vi "Untitled 1-save me.vi"() -> ()   [LabVIEW 2011]
uses:
  <vilib>/DAQmx/read.llb/DAQmx Read (Analog Wfm 1Chan NSamp).vi
  <vilib>/DAQmx/create/channels.llb/DAQmx Create Channel (AI-Current-Basic).vi
  <vilib>/DAQmx/configure/timing.llb/DAQmx Timing (Sample Clock).vi
  <vilib>/DAQmx/miscellaneous.llb/DAQmx Fill In Error Info.vi
  <vilib>/Analysis/NI_AALBase.lvlib
panel:
  in  "ECOLAB Button":bool=TRUE
  out "Max Value":dbl
  out "Maximum":string
  out "Block Count":i32
  in  "Tab Control":enum32{"DISPLAY", "CONFIG", "CALIBRATE"}(tab)
  in  "Intervals":i32=10
  in  "Rate (Inches / Second)":dbl
  out "XY Graph":cluster{dbl[], "Initialize Value":dbl[]}(graph)
  out "Histogram Graph":T1(graph)
  out "Save Error":errorcluster
  out "Distance Between Measurements (Inches)":dbl
  out "dt":dbl
  out "Main Error":errorcluster
  out "DAQ Error":errorcluster
  in  "DAQ Selection":tag
  in  "File Path Input":path
  in  "Samples/Channel":i32=5
  in  "Sample Rate (Hz)":dbl=500.0
  in  "Comments (Saves to Data File)":string
  in  "Scale Template":T2={"Channel Select"=0, "Clear/Reset Scales"=FALSE, "Channel #"=["0", "1", "2"], "Scale Names"=["a", "b", "c"], "Set?"=[FALSE, FALSE, FALSE, FALSE, FALSE, FALSE], "HI/LO Setpoints"=[1.0, 0.0, 1.0, 0.0, 1.0, 0.0], "Units"=["vdc", "vdc", "vdc"], "HI/LO Signals"=[1.0, 0.0, 1.0, 0.0, 1.0, 0.0], "Slope/Intercept"=[1.0, 0.0, 1.0, 0.0, 1.0, 0.0], "IN/OUT Values"=[1.0, 1.0, 2.0, 2.0, 3.0, 3.0]} {"Channel Select" min=0 step=1; "Slope/Intercept" format="%#.3p"; "HI/LO Setpoints" format="%#.3p"; "IN/OUT Values" format="%#.3p"; "HI/LO Signals" format="%#.3p"}
  in  "Simulate Signal?":bool
  in  "Simulated Signal":dbl
  in  "Stop Program":bool
  out "Measurements 2":string[](array[string])
  in  "Analyze Data?":bool
  in  "Reset Block Count?":bool
  in  "Update Rate [ms] 2":u32
  out "DAQ Loop":i32
  in  "Distance Threshold (> = Measure)":dbl
  in  "Save Data Signal":bool
  in  "Update Rate [ms]":u32
  in  "Input Signal":dbl
  in  "Flow Volume":dbl
  in  "Reset Spray Count":bool
  out "Spray Count":i32
  out "Temperature OUT":cluster{"Mean":dbl, "Stdev":dbl, "Max":dbl}
  out "output array":dbl[](array[numeric])
  out "Flow Delta":dbl
  out "loop":i32
  in  "stop":bool
  in  "Spray Signal":bool=TRUE
  # "Threshold (inches)"
  # "Block Count"
  # "Maximum (inches)"
  # "Block Profile Measurement Program"
  # "Blake Otting - 2011"
  # "Histogram of Maximum Value Measurements"
  # "Measurement Profile of Last Block"
  # "Track Rate"
  # "Inches / Second"
  # "Ch.\n#"
  # "Scale\nName"
  # "Set\nValues?"
  # "Scaled"
  # "Pre-Scaled"
  # "Scaling Result"
  # "Values"
  # "Units"
  # "Values"
  # "Channel\nSelect"
  # "HI"
  # "Slope"
  # "IN"
  # "LO"
  # "Intercept"
  # "OUT"
  # "HI"
  # "Slope"
  # "IN"
  # "LO"
  # "Intercept"
  # "OUT"
  # "HI"
  # "Slope"
  # "IN"
  # "LO"
  # "Intercept"
  # "OUT"
  # "HI"
  # "Slope"
  # "IN"
  # "LO"
  # "Intercept"
  # "OUT"
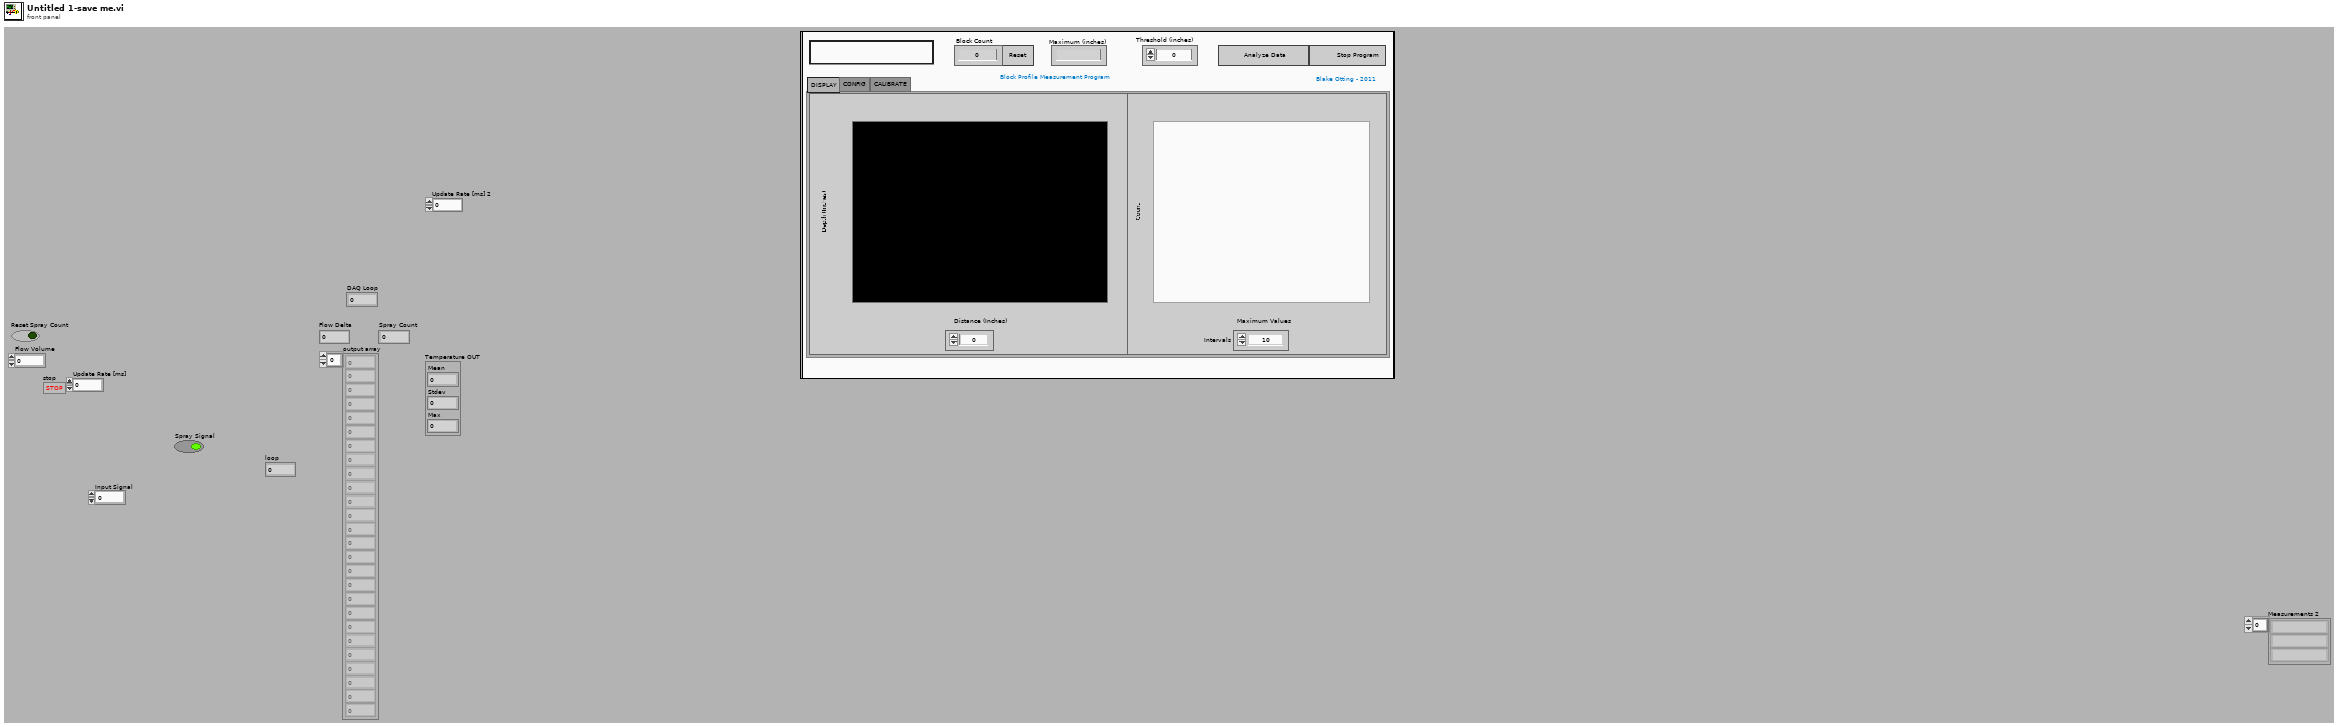
[diagram p1: front panel]
types:
  T1 = cluster{"X Values":dbl[], "Histogram: h(x)":i32[]}
  T2 = cluster{"Channel Select":i32, "Clear/Reset Scales":bool, "Channel #":string[], "Scale Names":string[], "Set?":bool[], "HI/LO Setpoints":dbl[], "Units":string[], "HI/LO Signals":dbl[], "Slope/Intercept":dbl[], "IN/OUT Values":dbl[]}
  T3 = cluster{"Delta":dbl, "Mean":dbl, "Stdev":dbl, "Max":dbl}
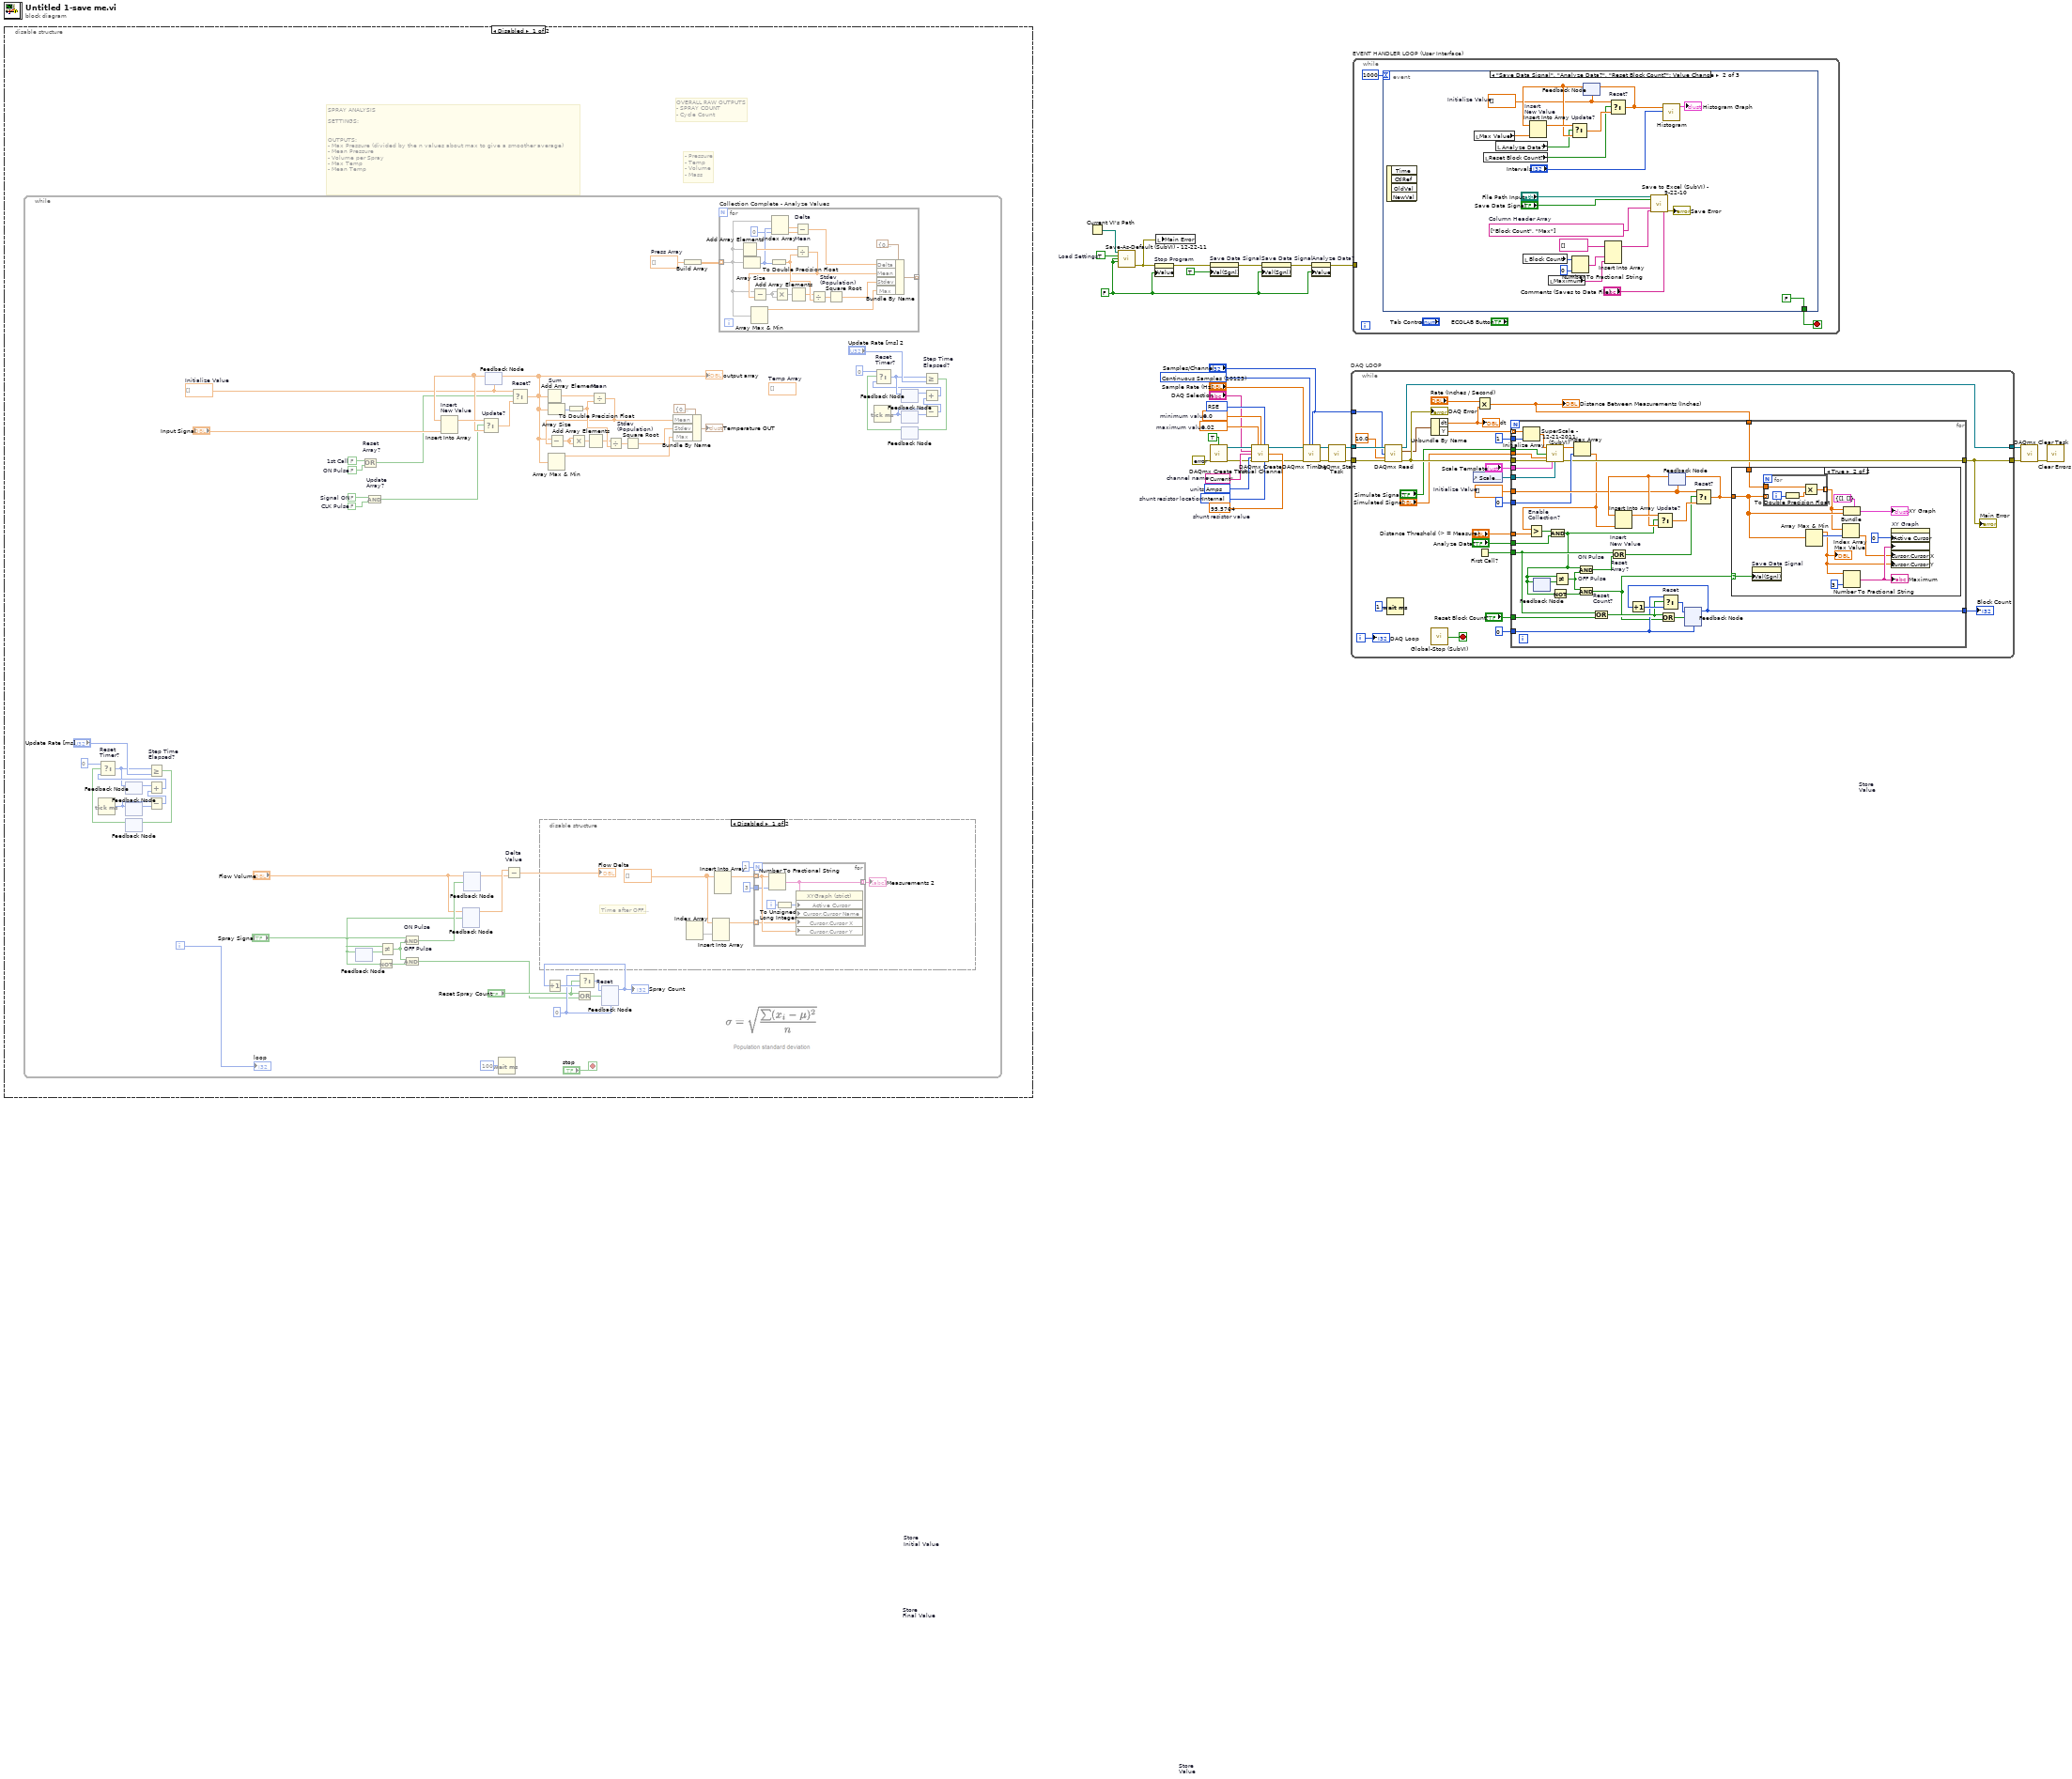
[diagram p0: block diagram]
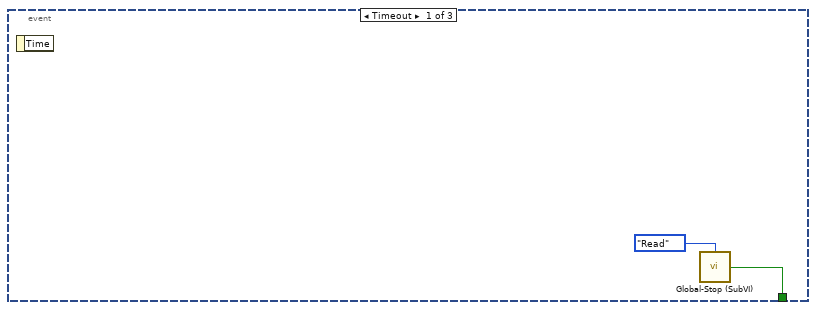
[diagram p2: hidden frame]
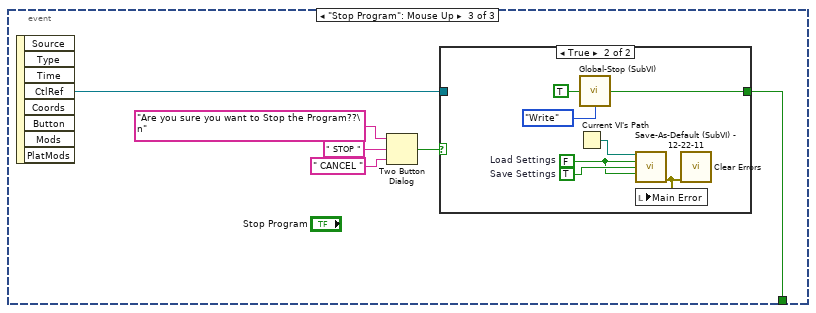
[diagram p3: hidden frame]
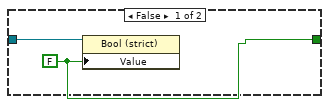
[diagram p4: hidden frame]
diagram:
  w5 = TRUE  # Load Settings
  w3 = FALSE
  w17 = 10123 items=["Finite Samples"=10178, "Continuous Samples"=10123, "Hardware Timed Single Point"=12522] ("Sample Mode")
  w25 = 10083 items=["default"=-1, "RSE"=10083, "NRSE"=10078, "Differential"=10106, "Pseudodifferential"=12529]
  w26 = 10342 items=["Amps"=10342, "From Custom Scale"=10065]  # units
  w27 = 95.5764  # shunt resistor value
  w28 = 10200 items=["Internal"=10200, "External"=10167]  # shunt resistor location
  w29 = "Current"  # channel name
  w30 = 0.0  # minimum value
  w31 = 0.02  # maximum value
  n1 = disable-structure shown="Disabled" {
    frame Disabled {
      # "- Pressure\n- Temp\n- Volume\n- Mass"
      # "OVERALL RAW OUTPUTS\n- SPRAY COUNT\n- Cycle Count"
      # "SPRAY ANALYSIS\n\nSETTINGS:\n\n\nOUTPUTS:\n- Max Pressure (divided by the n values about max to give a smoother average)\n- Mean Pressure\n- Volume per Spray \n- Max Temp\n- Mean Temp"
      n2 = while {
        i -> [w90]
        stop <- "stop" stop-if-true
        w46 = FALSE  # CLK Pulse
        w47 = FALSE  # Signal ON
        w49 = FALSE  # ON Pulse
        w50 = FALSE  # 1st Call
        w62 = dbl[] []  # Initialize Value
        w71 = 0 ("index")
        w75 = dbl[] []  # Press Array
        (unwired) dbl[] []  # Temp Array
        # "Time after OFF..."
        n3 = Tick Count (ms)() -> (millisecond timer value=w58:u32)
        n4 = feedback #1() -> (w59:u32)  [unwired: 1 in]
        n5 = feedback #2() -> (w57:u32)  [unwired: 1 in]
        n6 = feedback-in #2(w58) -> ()
        n7 = feedback #3() -> (w52:bool)  [unwired: 1 in]
        n8 = Subtract(x=w58, y=w57) -> (x-y=w55:u32)
        n9 = Add(x=w59, y=w55) -> (x+y=w60:u32)
        n10 = Select "Reset\nTimer?"(t=u32 0 ("x+y"), s=w52, f=w60) -> (s? t:f=w51:u32)
        n11 = feedback-in #1(w51) -> ()
        n12 = Greater Or Equal? "Step Time\nElapsed?"(x=w51, y="Update Rate [ms]") -> (x >= y?=w53:bool)
        n13 = feedback-in #3(w53) -> ()
        n14 = feedback #4() -> (w98:bool)  [unwired: 1 in]
        n15 = feedback-in #4("Spray Signal") -> ()
        n16 = Or "Reset\nArray?"(x=w50, y=w49) -> (x .or. y?=w48:bool)
        n17 = And "Update\nArray?"(x=w47, y=w46) -> (x .and. y?=w45:bool)
        n18 = Not(x="Spray Signal") -> (.not. x?=w94:bool)
        n19 = Not Equal?(x="Spray Signal", y=w98) -> (x != y?=w95:bool)
        n20 = And "ON Pulse"(x="Spray Signal", y=w95) -> (x .and. y?=w89:bool)
        n21 = And "OFF Pulse"(x=w95, y=w94) -> (x .and. y?=w67:bool)
        n22 = feedback #5 "Store \nFinal Value"() -> (w93:dbl)  [unwired: 1 in]
        n23 = feedback-in #5("Flow Volume", "Spray Signal") -> ()
        n24 = feedback #6 "Store \nInitial Value"() -> (w92:dbl)  [unwired: 1 in]
        n25 = feedback-in #6("Flow Volume", w89) -> ()
        n26 = feedback #7(w62) -> (w64:dbl[])
        n27 = Insert Into Array "Insert \nNew Value"(array=w64, new element="Input Signal") -> (w65:dbl[])  [unwired: 1 in]
        n28 = Select "Update?"(t=w65, s=w45, f=w64) -> (s? t:f=w63:dbl[])
        n29 = Wait (ms)(milliseconds to wait=u32 100) -> ()  [unwired: 1 out]
        n30 = Subtract "Delta\nValue"(x=w93, y=w92) -> (x-y=→"Flow Delta":dbl)
        n31 = Select "Reset?"(t=w62, s=w48, f=w63) -> (s? t:f=w44:dbl[])
        "output array" <- w44
        n32 = feedback-in #7(w44) -> ()
        n33 = disable-structure shown="Disabled" {
          frame Disabled {
            w104 = dbl[] [] ("appended array")
            n34 = Index Array() -> (element #1=w105, index #1=w110:i32, element #2=w103, index #2=w109:i32)  [unwired: 1 in]
            n35 = Insert Into Array(array=w104, new element #1=w105, new element #2=w103) -> (w102:dbl[])  [unwired: 1 in]
            n36 = Insert Into Array(array=w104) -> (w107:dbl[], new element #1=w108:dbl, new element #2=w106:dbl)  [unwired: 1 in]
            n37 = for {
              N: 1 -> [_]
              tunnel: [w114] -> w99 mode=indexing
              tunnel: w107 -> [w113] mode=indexing
              tunnel: w102 -> [w112] mode=indexing
              tunnel: i16 3 ("precision (6)") -> [w111]
              i -> [w115]
              n38 = Number To Fractional String(number=w113, precision (6)=w111) -> (F-format string=w114:string)  [unwired: 2 in]
              n39 = To Unsigned Long Integer(number=w115) -> (unsigned 32bit integer=w116:u32)
              n40 = property on="Property Node" class="XYGraph (strict)"("Active Cursor"=w116, "Cursor.Cursor Name"=w114, "Cursor.Cursor X"=w112, "Cursor.Cursor Y"=w113) -> ()  [unwired: 2 in, 2 out]
            }
            "Measurements 2" <- w99
          }
          frame Enabled {
          }
        }
        n41 = Add Array Elements "Sum"(numeric array=w44) -> (sum=w87:dbl)
        n42 = Array Size(array=w44) -> (size(s)=w86:i32)
        n43 = Array Max & Min(array=w44) -> (max value=w78:dbl)  [unwired: 3 out]
        n44 = To Double Precision Float(number=w86) -> (double precision float=w83:dbl)
        n45 = Or(x="Reset Spray Count", y=w67) -> (x .or. y?=w68:bool)
        n46 = Divide "Mean"(x=w87, y=w83) -> (x/y=w77:dbl)
        n47 = Subtract(x=w44, y=w77) -> (x-y=w85:dbl[])
        n48 = Multiply(x=w85, y=w85) -> (x*y=w84:dbl[])
        n49 = Add Array Elements(numeric array=w84) -> (sum=w82:dbl)
        n50 = feedback #8 "Store\nValue"(w71) -> (w73:i32)
        "Spray Count" <- w73
        n51 = Increment(x=w73) -> (x+1=w72:i32)
        n52 = Select "Reset"(t=w71, s="Reset Spray Count", f=w72) -> (s? t:f=w70:i32)
        n53 = feedback-in #8(w70, w68) -> ()
        n54 = Divide(x=w82, y=w83) -> (x/y=w81:dbl)
        n55 = Square Root "Stdev\n(Population)"(x=w81) -> (sqrt(x)=w79:dbl)
        n56 = Bundle By Name(cluster=cluster{"Mean":dbl, "Stdev":dbl, "Max":dbl} {"Mean"=0.0, "Stdev"=0.0, "Max"=0.0}, "Mean"=w77, "Stdev"=w79, "Max"=w78) -> (→"Temperature OUT":cluster{"Mean":dbl, "Stdev":dbl, "Max":dbl})
        n57 = Build Array(w75) -> (w74:dbl[][])
        n58 = for "Collection Complete - Analyze Values" {
          tunnel: w74 -> [w118] mode=indexing
          tunnel: [w117] -> _ mode=indexing
          n59 = Add Array Elements(numeric array=w118) -> (sum=w133:dbl)
          n60 = Array Size(array=w118) -> (size(s)=w123:i32)
          n61 = Array Max & Min(array=w118) -> (max value=w125:dbl)  [unwired: 3 out]
          n62 = To Double Precision Float(number=w123) -> (double precision float=w130:dbl)
          n63 = Index Array(array=w118, index #1=w123, index #2=0 ("index")) -> (element #1=w120:dbl, element #2=w121:dbl)
          n64 = Subtract "Delta"(x=w120, y=w121) -> (x-y=w119:dbl)
          n65 = Divide "Mean"(x=w133, y=w130) -> (x/y=w124:dbl)
          n66 = Subtract(x=w118, y=w124) -> (x-y=w132:dbl[])
          n67 = Multiply(x=w132, y=w132) -> (x*y=w131:dbl[])
          n68 = Add Array Elements(numeric array=w131) -> (sum=w129:dbl)
          n69 = Divide(x=w129, y=w130) -> (x/y=w128:dbl)
          n70 = Square Root "Stdev\n(Population)"(x=w128) -> (sqrt(x)=w126:dbl)
          n71 = Bundle By Name(cluster=T3 {"Delta"=0.0, "Mean"=0.0, "Stdev"=0.0, "Max"=0.0}, "Delta"=w119, "Mean"=w124, "Stdev"=w126, "Max"=w125) -> (w117:T3)
        }
        n72 = Tick Count (ms)() -> (millisecond timer value=w42:u32)
        n73 = feedback #9() -> (w43:u32)  [unwired: 1 in]
        n74 = feedback #10() -> (w41:u32)  [unwired: 1 in]
        n75 = feedback-in #10(w42) -> ()
        n76 = feedback #11() -> (w36:bool)  [unwired: 1 in]
        n77 = Subtract(x=w42, y=w41) -> (x-y=w39:u32)
        n78 = Add(x=w43, y=w39) -> (x+y=w34:u32)
        n79 = Select "Reset\nTimer?"(t=u32 0 ("x+y"), s=w36, f=w34) -> (s? t:f=w35:u32)
        n80 = feedback-in #9(w35) -> ()
        n81 = Greater Or Equal? "Step Time\nElapsed?"(x=w35, y="Update Rate [ms] 2") -> (x >= y?=w37:bool)
        n82 = feedback-in #11(w37) -> ()
        "loop" <- w90
      }
    }
    frame Enabled {
    }
  }
  n83 = Current VI's Path() -> (path=w6:path)
  n84 = call "Save-As-Default (SubVI) - 12-22-11.vi"("Current VI's Path"=w6, "Load Settings"=w5, "Save Settings"=w3, "Save and Exit"=w3) -> ("Error Output"=w4:errorcluster)  [unwired: 11 in]
  n85 = property on="Stop Program" class="Bool (strict)"(error in=w4, "Value"=w3) -> (error out=w7:errorcluster)  [unwired: 1 in, 1 out]
  n86 = local write "Main Error"(w4) -> ()
  n87 = property on="Save Data Signal" class="Bool (strict)"(error in=w7, "Val(Sgnl)"=TRUE) -> (error out=w8:errorcluster)  [unwired: 1 in, 1 out]
  n88 = call <vilib>:"DAQmx Create Task.vi"("auto cleanup"=TRUE, "error in"=errorcluster {"status"=FALSE, "code"=0, "source"=""}) -> ("task out"=w24:refnum<k21>, "error out"=w23:errorcluster)  [unwired: 12 in]
  n89 = call-poly <vilib>:"DAQmx Create Virtual Channel.vi"("task in"=w24, "maximum value"=w31, "minimum value"=w30, "input terminal configuration"=w25, "physical channels"="DAQ Selection", "name to assign"=w29, "external shunt resistor value"=w27, "units"=w26, "error in"=w23, "shunt resistor location"=w28) -> ("task out"=w16:refnum<k21>, "error out"=w15:errorcluster)  [unwired: 1 in, 3 out]
  n90 = property on="Save Data Signal" class="Bool (strict)"(error in=w8, "Val(Sgnl)"=w3) -> (error out=w2:errorcluster)  [unwired: 1 in, 1 out]
  n91 = call-poly <vilib>:"DAQmx Timing.vi"("task/channels in"=w16, "sample mode"=w17, "samples per channel"="Samples/Channel", "rate"="Sample Rate (Hz)", "error in"=w15) -> ("task out"=w13:refnum<k21>, "error out"=w14:errorcluster)  [unwired: 2 in, 7 out]
  n92 = property on="Analyze Data?" class="Bool (strict)"(error in=w2, "Value"=w3) -> (error out=w1:errorcluster)  [unwired: 1 in, 1 out]
  n93 = call <vilib>:"DAQmx Start Task.vi"("task/channels in"=w13, "error in"=w14) -> ("task out"=w12:refnum<k21>, "error out"=w11:errorcluster)  [unwired: 12 in]
  n94 = while "DAQ LOOP" {
    tunnel: [w134] -> w32
    tunnel: w11 -> [w147]
    tunnel: w12 -> [w148]
    tunnel: [w138] -> w19
    tunnel: "Samples/Channel" -> [w146]
    i -> [w161]
    stop <- w139 stop-if-true
    w149 = dbl[] []  # Initialize Value
    n95 = call-poly <vilib>:"DAQmx Read.vi"("task/channels in"=w148, "number of samples per channel"=w146, "timeout"=10.0, "error in"=w147) -> ("task out"=w134:refnum<k21>, "data"=w143:waveform(dbl), "error out"=w144:errorcluster)  [unwired: 9 in]
    "DAQ Error" <- w144
    n96 = Wait (ms)(milliseconds to wait=u32 1) -> ()  [unwired: 1 out]
    n97 = Unbundle By Name(w143) -> ("dt"=w141:dbl, "Y"=w142:dbl[])
    "dt" <- w141
    n98 = call "Global-Stop (SubVI).vi"() -> ("OUT"=w139:bool)  [unwired: 4 in]
    n99 = control-ref of="Scale Template"() -> (w155:refnum<vi>)
    n100 = Multiply(x="Rate (Inches / Second)", y=w141) -> (x*y=w135:dbl)
    "Distance Between Measurements (Inches)" <- w135
    n101 = First Call?() -> (First Call?: T/F=w153:bool)
    n102 = for {
      tunnel: w142 -> [w197] mode=indexing
      tunnel: "Distance Threshold (> = Measure)" -> [w165]
      tunnel: "Analyze Data?" -> [w181]
      tunnel: w149 -> [w180]
      tunnel: 1 ("dimension size") -> [w178]
      tunnel: 0 ("index") -> [w177]
      tunnel: 0 ("index") -> [w176]
      tunnel: w153 -> [w175]
      tunnel: "Reset Block Count?" -> [w174]
      tunnel: [w173] -> w138
      tunnel: w144 -> [w172]
      tunnel: "Scale Template" -> [w171]
      tunnel: w155 -> [w170]
      tunnel: [w167] -> w156
      tunnel: w135 -> [w168]
      tunnel: "Simulate Signal?" -> [w164]
      tunnel: "Simulated Signal" -> [w163]
      n103 = Initialize Array(w197, w178) -> (w196:dbl[])
      n104 = feedback #12() -> (w189:bool)  [unwired: 1 in]
      n105 = call "SuperScale - 12-21-2011 (SubVI).vi"("Measured Signals"=w196, "Simulate Signal?"=w164, "Simulated Signal"=w163, "Error Input"=w172, "Scale Template"=w171, "Scale Ref"=w170) -> ("Scaled Values"=w195:dbl[], "Scale Error"=w173:errorcluster)  [unwired: 8 in]
      n106 = Index Array(array=w195, index=w177) -> (element=w169:dbl)
      n107 = Greater? "Enable\nCollection?"(x=w169, y=w165) -> (0:w194:bool)
      n108 = And(x=w194, y=w181) -> (x .and. y?=w162:bool)
      n109 = feedback-in #12(w162) -> ()
      n110 = Not(x=w162) -> (.not. x?=w187:bool)
      n111 = Not Equal?(x=w162, y=w189) -> (x != y?=w188:bool)
      n112 = And "ON Pulse"(x=w162, y=w188) -> (x .and. y?=w183:bool)
      n113 = And "OFF Pulse"(x=w188, y=w187) -> (x .and. y?=w166:bool)
      n114 = Or "Reset\nCount?"(x=w175, y=w174) -> (x .or. y?=w182:bool)
      n115 = Or "Reset\nArray?"(x=w175, y=w183) -> (x .or. y?=w190:bool)
      n116 = Or(x=w182, y=w166) -> (x .or. y?=w184:bool)
      n117 = feedback #13(w180) -> (w192:dbl[])
      n118 = Insert Into Array "Insert \nNew Value"(array=w192, new element=w169) -> (w193:dbl[])  [unwired: 1 in]
      n119 = Select "Update?"(t=w193, s=w162, f=w192) -> (s? t:f=w191:dbl[])
      n120 = feedback #14 "Store\nValue"(w176) -> (w167:i32)
      n121 = Increment(x=w167) -> (x+1=w186:i32)
      n122 = Select "Reset"(t=w176, s=w182, f=w186) -> (s? t:f=w185:i32)
      n123 = feedback-in #14(w185, w184) -> ()
      n124 = Select "Reset?"(t=w180, s=w190, f=w191) -> (s? t:f=w179:dbl[])
      n125 = feedback-in #13(w179) -> ()
      n126 = case shown="True" w166 {
        selector: w166 -> [_ w198]
        tunnel: w179 -> [_ w208]
        tunnel: w168 -> [_ w209]
        frame False {
        }
        frame True {
          n127 = property on="Save Data Signal" class="Bool (strict)"("Val(Sgnl)"=w198) -> ()  [unwired: 2 in, 2 out]
          n128 = for {
            tunnel: w208 -> [_] mode=indexing
            tunnel: w209 -> [w213]
            tunnel: [w210] -> w206 mode=indexing
            i -> [w211]
            n129 = To Double Precision Float(number=w211) -> (double precision float=w212:dbl)
            n130 = Multiply(x=w213, y=w212) -> (x*y=w210:dbl)
          }
          n131 = Array Max & Min(array=w208) -> (max value=w200:dbl, max index (indices)=w205:i32)  [unwired: 2 out]
          "Max Value" <- w200
          n132 = Index Array(array=w206, index=w205) -> (element=w201:dbl)
          n133 = Bundle(cluster=cluster{dbl[], "Initialize Value":dbl[]} {[], "Initialize Value"=[]}, w206, "Initialize Value"=w208) -> (→"XY Graph":cluster{dbl[], "Initialize Value":dbl[]})
          n134 = Number To Fractional String(number=w200, precision (6)=i16 3) -> (F-format string=w202:string)  [unwired: 2 in]
          "Maximum" <- w202
          n135 = property on="XY Graph" class="XYGraph (strict)"("Active Cursor"=u32 0, "Cursor.Cursor Name"=w202, "Cursor.Cursor X"=w201, "Cursor.Cursor Y"=w200) -> ()  [unwired: 2 in, 2 out]
        }
      }
    }
    "Block Count" <- w156
    "Main Error" <- w138
    "DAQ Loop" <- w161
  }
  n136 = while "EVENT HANDLER LOOP (User Interface)" {
    tunnel: w1 -> [_]
    stop <- w215 stop-if-true
    n137 = event shown="[1] \"Save Data Signal\", \"Analyze Data?\", \"Reset Block Count?\": Value Change" {
      selector: _ -> [_ _ _]
      dyn-events: _ -> [_ _ _]
      timeout: 1000 -> [_ _ _]
      tunnel: [w216 FALSE ("OUT") w241] -> w215
      event Timeout {
        n138 = event-data() -> ()  [unwired: 2 out]
        n139 = call "Global-Stop (SubVI).vi"("Mode (Read)"=enum16{"Read", "Write"}."Read") -> ("OUT"=w216:bool)  [unwired: 3 in]
      }
      event "Save Data Signal", "Analyze Data?", "Reset Block Count?": Value Change {
        w222 = string[] ["Block Count", "Max"]  # Column Header Array
        w235 = dbl[] []  # Initialize Value
        n140 = event-data() -> ()  [unwired: 5 out]
        n141 = local read "Max Value"() -> (w232:dbl)
        n142 = local read "Reset Block Count?"() -> (w234:bool)
        n143 = local read "Analyze Data?"() -> (w233:bool)
        n144 = local read "Block Count"() -> (w226:i32)
        n145 = local read "Maximum"() -> (w219:string)
        n146 = Number To Fractional String(number=w226, precision (6)=i16 0) -> (F-format string=w227:string)  [unwired: 2 in]
        n147 = feedback #15(w235) -> (w237:dbl[])
        n148 = Insert Into Array "Insert \nNew Value"(array=w237, new element=w232) -> (w238:dbl[])  [unwired: 1 in]
        n149 = Select "Update?"(t=w238, s=w233, f=w237) -> (s? t:f=w236:dbl[])
        n150 = Insert Into Array(array=string[] [] ("F-format string"), new element #1=w227, new element #2=w219) -> (w223:string[])  [unwired: 1 in]
        n151 = Select "Reset?"(t=w235, s=w234, f=w236) -> (s? t:f=w231:dbl[])
        n152 = feedback-in #15(w231) -> ()
        n153 = call "Save to Excel (SubVI) - 9-22-10.vi"("File Path Input"="File Path Input", "Save (Enable/Signal)"="Save Data Signal", "Column Header Array"=w222, "Data Array (Row)"=w223, "Comments"="Comments (Saves to Data File)") -> ("Error Output"=→"Save Error":errorcluster)  [unwired: 10 in, 4 out]
        n154 = call <vilib>:"Histogram.vi"("intervals"="Intervals", "X"=w231) -> ("Histogram Graph"=→"Histogram Graph":T1)  [unwired: 6 in, 3 out]
      }
      event "Stop Program": Mouse Up {
        n155 = event-data() -> ("CtlRef"=w240:refnum<vi>)  [unwired: 8 out]
        n156 = Two Button Dialog(message="Are you sure you want to Stop the Program??\n", 1:" CANCEL " ("F button name (\"Cancel\")"), 2:" STOP ") -> (T button?=w242:bool)
        n157 = case shown="True" w242 {
          tunnel: [w246 w252] -> w241
          tunnel: w240 -> [w247 _]
          frame False {
            w246 = FALSE ("Value")
            n158 = property class="Bool (strict)"(reference=w247, "Value"=w246) -> ()  [unwired: 1 in, 2 out]
          }
          frame True {
            w250 = TRUE  # Save Settings
            w249 = FALSE  # Load Settings
            n159 = Current VI's Path() -> (path=w251:path)
            n160 = call "Global-Stop (SubVI).vi"("Mode (Read)"=enum16{"Read", "Write"}."Write", "IN"=TRUE) -> ("OUT"=w252:bool)  [unwired: 2 in]
            n161 = call "Save-As-Default (SubVI) - 12-22-11.vi"("Current VI's Path"=w251, "Load Settings"=w249, "Save Settings"=w250, "Save and Exit"=w249) -> ("Error Output"=w248:errorcluster)  [unwired: 11 in]
            n162 = local write "Main Error"(w248) -> ()
            n163 = call <vilib>:"Clear Errors.vi"("error in (no error)"=w248) -> ()  [unwired: 7 out]
          }
        }
      }
    }
  }
  n164 = call <vilib>:"DAQmx Clear Task.vi"("task in"=w32, "error in"=w19) -> ("error out"=w33:errorcluster)  [unwired: 13 out]
  n165 = call <vilib>:"Clear Errors.vi"("error in (no error)"=w33) -> ()  [unwired: 6 in, 1 out]
